vi "Wrap_Baudrate.vi"(8 "BTR0BTR1(User)":i16 format="%.0x", 9 "Wrap numeric Baudrate to ENUM":bool, 10 "TPCANBaudrate numeric":u16, 11 "TPCANBaudrate ENUM":T1) -> (2 "TPCANBaudrate ENUM out":T1, 3 "Numeric out":u16)   [LabVIEW 2016]
doc: "Wrap the ENUM Baudrate to a numeric value and vice versa"
uses:
  <instrlib>/KDI Digital Instrumentation/API_for_PCAN_BASIC_FD/TPCANBaudrate.ctl
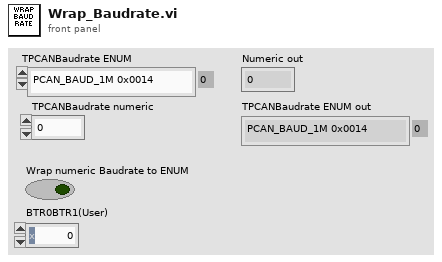
[diagram p1: front panel]
types:
  T1 = typedef "TPCANBaudrate.ctl" = enum16{"PCAN_BAUD_1M 0x0014", "PCAN_BAUD_800K 0x0016", "PCAN_BAUD_500K 0x001C", "PCAN_BAUD_250K 0x011C", "PCAN_BAUD_125K 0x031C", "PCAN_BAUD_100K 0x432F", "PCAN_BAUD_95K 0xC34E", "PCAN_BAUD_83K 0x852B", "PCAN_BAUD_50K 0x472F", "PCAN_BAUD_47K 0x1414", "PCAN_BAUD_33K 0x8B2F", "PCAN_BAUD_20K 0x532F", "PCAN_BAUD_10K 0x672F", "PCAN_BAUD_5K 0x7F7F", "User Baudrate"}
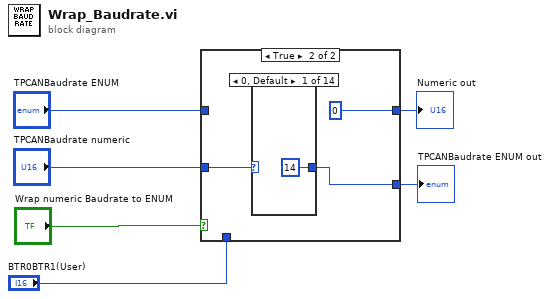
[diagram p0: block diagram]
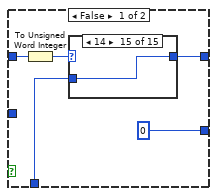
[diagram p2: hidden frame]
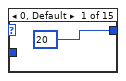
[diagram p3: hidden frame]
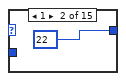
[diagram p4: hidden frame]
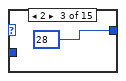
[diagram p5: hidden frame]
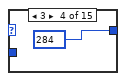
[diagram p6: hidden frame]
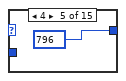
[diagram p7: hidden frame]
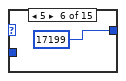
[diagram p8: hidden frame]
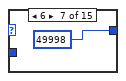
[diagram p9: hidden frame]
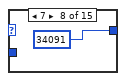
[diagram p10: hidden frame]
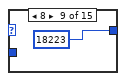
[diagram p11: hidden frame]
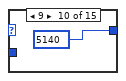
[diagram p12: hidden frame]
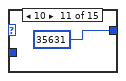
[diagram p13: hidden frame]
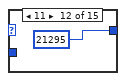
[diagram p14: hidden frame]
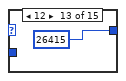
[diagram p15: hidden frame]
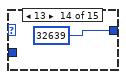
[diagram p16: hidden frame]
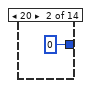
[diagram p17: hidden frame]
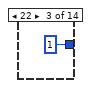
[diagram p18: hidden frame]
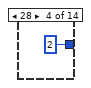
[diagram p19: hidden frame]
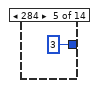
[diagram p20: hidden frame]
diagram:
  n1 = case shown="True" "Wrap numeric Baudrate to ENUM" {
    tunnel: [w11 u16 0] -> w6
    tunnel: "TPCANBaudrate ENUM" -> [w9 _]
    tunnel: "TPCANBaudrate numeric" -> [_ w28]
    tunnel: [0 w27] -> w2
    tunnel: "BTR0BTR1(User)" -> [w7 _]
    frame False {
      n2 = To Unsigned Word Integer(number=w9) -> (unsigned 16bit integer=w10:u16)
      n3 = case shown="14" w10 {
        tunnel: [u16 20 u16 22 u16 28 u16 284 u16 796 u16 17199 u16 49998 u16 34091 u16 18223 u16 5140 u16 35631 u16 21295 u16 26415 u16 32639 w26] -> w11
        tunnel: w7 -> [_ _ _ _ _ _ _ _ _ _ _ _ _ _ w26]
        frame 0, Default {
        }
        frame 1 {
        }
        frame 2 {
        }
        frame 3 {
        }
        frame 4 {
        }
        frame 5 {
        }
        frame 6 {
        }
        frame 7 {
        }
        frame 8 {
        }
        frame 9 {
        }
        frame 10 {
        }
        frame 11 {
        }
        frame 12 {
        }
        frame 13 {
        }
        frame 14 {
        }
      }
    }
    frame True {
      n4 = case shown="0, Default" w28 {
        tunnel: [u16 14 ("TPCANBaudrate numeric") u16 0 ("TPCANBaudrate numeric") u16 1 ("TPCANBaudrate numeric") u16 2 ("TPCANBaudrate numeric") u16 3 ("TPCANBaudrate numeric") u16 4 ("TPCANBaudrate numeric") u16 5 ("TPCANBaudrate numeric") u16 6 ("TPCANBaudrate numeric") u16 7 ("TPCANBaudrate numeric") u16 8 ("TPCANBaudrate numeric") u16 10 ("TPCANBaudrate numeric") u16 11 ("TPCANBaudrate numeric") u16 12 ("TPCANBaudrate numeric") u16 13 ("TPCANBaudrate numeric")] -> w27
        frame 0, Default {
        }
        frame 20 {
        }
        frame 22 {
        }
        frame 28 {
        }
        frame 284 {
        }
        frame 796 {
        }
        frame 17199 {
        }
        frame 49998 {
        }
        frame 34088 {
        }
        frame 18223 {
        }
        frame 34863 {
        }
        frame 21295 {
        }
        frame 26415 {
        }
        frame 32639 {
        }
      }
    }
  }
  "Numeric out" <- w6
  "TPCANBaudrate ENUM out" <- w2
